vi "sendReqstToTask.vi"(8 "error in (no error)":errorcluster, 9 "Parameter":variant, 10 "request":string, 11 "TaskRef in":refnum<vi>) -> (0 "error IO":errorcluster, 3 "TaskRef out":refnum<vi>)   [LabVIEW 2015, in "pdbm_task_route.lvlib"]
uses:
  pdbm_task_route.lvlib
  UsrDefine/TaskFeedbackCmd.ctl
  UsrDefine/TaskReqst.ctl
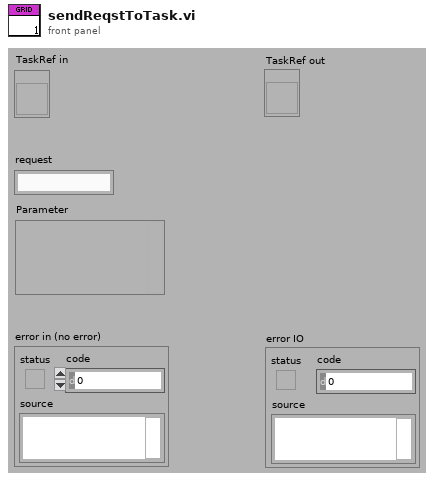
[diagram p1: front panel]
types:
  T1 = typedef "pdbm_task_route.lvlib/TaskReqst.ctl" = cluster{"Command":string, "Variant":variant}
  T2 = cluster{"pdbm_taskroute_feedback_event":refnum<user-event>, "pdbm_task_reqst_event":refnum<user-event>, "pdbm_testsystem_data":variant}
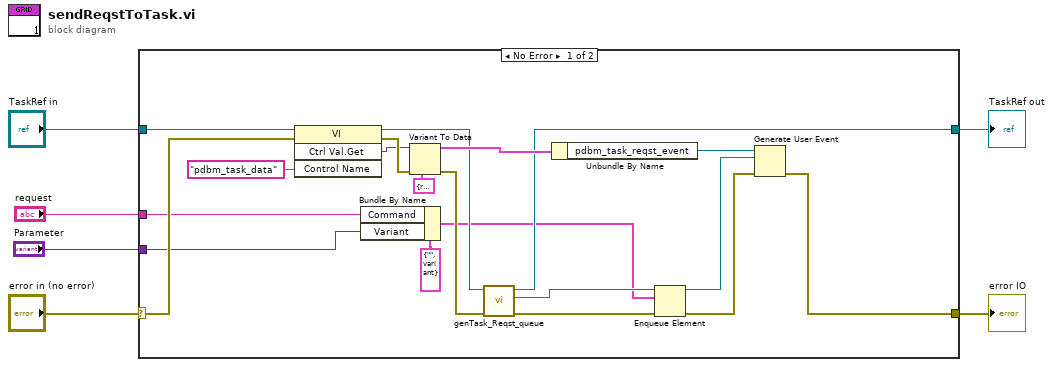
[diagram p0: block diagram]
diagram:
  n1 = case shown="No Error" "error in (no error)" {
    selector: "error in (no error)" -> [w25 w28]
    tunnel: "TaskRef in" -> [w26 w27]
    tunnel: [w13 w27] -> w2
    tunnel: [w7 w28] -> w1
    tunnel: "request" -> [w11 _]
    tunnel: "Parameter" -> [w10 _]
    frame No Error {
      n2 = invoke class="VI" method="Ctrl Val.Get"(reference=w26, error in=w25, "Control Name"="pdbm_task_data") -> (reference out=w14:refnum<vi>, error out=w23:errorcluster, "Get Control Value Variant"=w22:variant)  [unwired: 1 in, 1 out]
      n3 = Bundle By Name(cluster=T1 {"Command"="", "Variant"=variant} ("element"), "Command"=w11, "Variant"=w10) -> (w9:T1)
      n4 = Variant To Data(error in=w23, type=T2 {"pdbm_taskroute_feedback_event"=refnum, "pdbm_task_reqst_event"=refnum, "pdbm_testsystem_data"=variant} ("output cluster"), Variant=w22) -> (data=w20:T2, error out=w18:errorcluster)
      n5 = call "genTask_Reqst_queue.vi"("error in (no error)"=w18, "TaskRef"=w14) -> ("error IO"=w17:errorcluster, "TaskReqst_queue"=w16:refnum<queue>, "TaskRef out"=w13:refnum<vi>)  [unwired: 7 in]
      n6 = Unbundle By Name(w20) -> ("pdbm_task_reqst_event"=w19:refnum<user-event>)
      n7 = Enqueue Element(queue=w16, element=w9, error in (no error)=w17) -> (queue out=w15:refnum<queue>, error out=w12:errorcluster)  [unwired: 1 in, 1 out]
      n8 = Generate User Event(user event=w19, event data cluster=w15, error in=w12) -> (error out=w7:errorcluster)  [unwired: 1 in, 1 out]
    }
    frame Error {
    }
  }
  "TaskRef out" <- w2
  "error IO" <- w1
